vi "Arm Control Loop.vi"(8 "error in (no error)":errorcluster) -> ()   [LabVIEW 2011]
uses:
  Apendage State.ctl
  <vilib>/Rock Robotics/WPI/Solenoid/WPI_SolenoidValue.ctl
  Robot Global Data.vi
  <vilib>/Rock Robotics/WPI/Solenoid/WPI_SolenoidSetEnum.vi
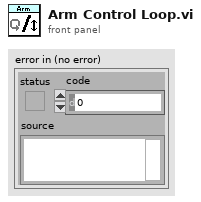
[diagram p1: front panel]
types:
  T1 = typedef "WPI_SolenoidValue.ctl" = enum16{"Off", "On", "Forward", "Reverse"}
  T2 = typedef "Apendage State.ctl" = enum16{"Unknown", "Down", "Up"}
  T3 = typedef "WPI_SolenoidDevRef.ctl" = cluster{"DevStatus":errorcluster, "Solenoid Module":T4, "Forward Solenoid Channel":T5, "Reverse Solenoid Channel":T5}
  T4 = typedef "FPGA_TypedefSolenoidModule.ctl" = enum16{"Solenoid Module 1", "Solenoid Module 2"}
  T5 = typedef "WPI_SolenoidChannel.ctl" = enum8{"Solenoid 1", "Solenoid 2", "Solenoid 3", "Solenoid 4", "Solenoid 5", "Solenoid 6", "Solenoid 7", "Solenoid 8", "Invalid"}
  T6 = typedef "WPI_RelayDevRef.ctl" = cluster{"DevStatus":errorcluster, "Relay Channel":T7, "Digital Module":T8, "Relay Direction":T9}
  T7 = typedef "FPGA_DIORelayChannel.ctl" = enum8{"Relay 1", "Relay 2", "Relay 3", "Relay 4", "Relay 5", "Relay 6", "Relay 7", "Relay 8", "Invalid"}
  T8 = typedef "FPGA_TypedefDigitalModule.ctl" = enum16{"Digital Module 1", "Digital Module 2"}
  T9 = typedef "WPI_RelayDirection.ctl" = enum16{"Both directions", "Forward only", "Reverse only"}
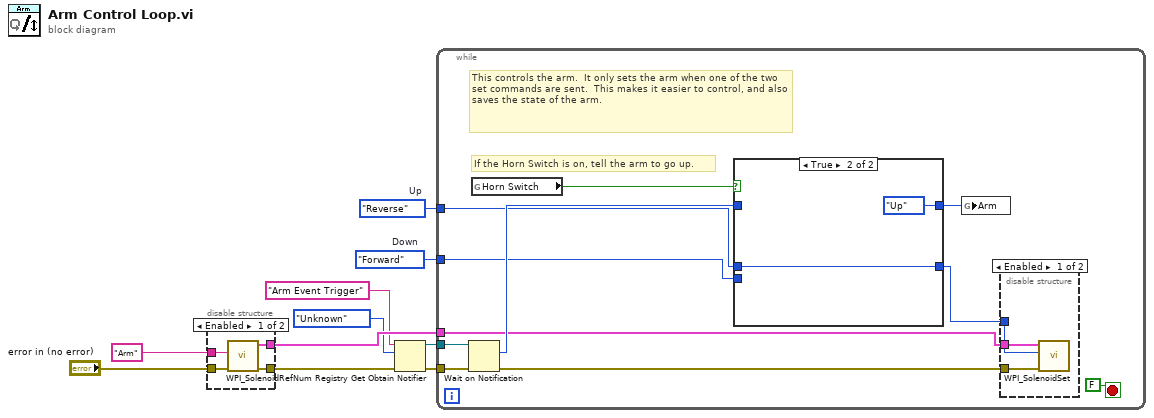
[diagram p0: block diagram]
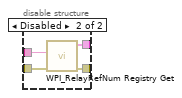
[diagram p2: hidden frame]
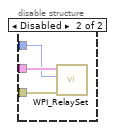
[diagram p3: hidden frame]
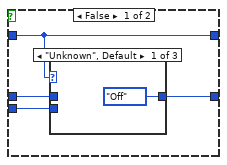
[diagram p4: hidden frame]
diagram:
  w1 = WPI_SolenoidValue."Forward"  # Down
  w2 = WPI_SolenoidValue."Reverse"  # Up
  n1 = disable-structure shown="Enabled" {
    disable-tunnel: [w14 w17] -> w8
    disable-tunnel: [w13 w18] -> w7
    disable-tunnel: "error in (no error)" -> [w12 w15]
    disable-tunnel: "Arm" ("refnum name") -> [w11 w16]
    frame Enabled {
      n2 = call <vilib>:"WPI_SolenoidRefNum Registry Get.vi"("error in (no error)"=w12, "refnum name"=w11) -> ("error out"=w13:errorcluster, "SolenoidDevRef"=w14:T3)  [unwired: 8 in]
    }
    frame Disabled {
      n3 = call <vilib>:"WPI_RelayRefNum Registry Get.vi"("error in (no error)"=w15, "refnum name"=w16) -> ("error out"=w18:errorcluster, "RelayDevRef"=w17:T6)  [unwired: 8 in]
    }
  }
  n4 = Obtain Notifier(name (unnamed)="Arm Event Trigger", notification data type=Apendage_State."Unknown", error in (no error)=w7) -> (notifier out=w10:refnum<notifier>, error out=w9:errorcluster)  [unwired: 1 in, 1 out]
  n5 = while {
    tunnel: w10 -> [w29]
    tunnel: w9 -> [w28]
    tunnel: w8 -> [w21]
    tunnel: w2 -> [w23]
    tunnel: w1 -> [w22]
    stop <- FALSE stop-if-true
    # "If the Horn Switch is on, tell the arm to go up."
    # "This controls the arm.  It only sets the arm when one of the two set commands are sent.  This makes it easier to control, and also saves the state of the arm."
    n6 = Wait on Notification(notifier=w29, error in (no error)=w28) -> (notification=w26:T2, error out=w19:errorcluster)  [unwired: 2 in, 2 out]
    n7 = global read "Robot Global Data.vi" "Horn Switch"() -> (w25:bool)
    n8 = case shown="True" w25 {
      tunnel: w26 -> [w39 _]
      tunnel: [w39 Apendage_State."Up"] -> w24
      tunnel: [w38 w43] -> w20
      tunnel: w23 -> [w37 w43]
      tunnel: w22 -> [w36 _]
      frame False {
        n9 = case shown="\"Unknown\", Default" w39 {
          tunnel: [WPI_SolenoidValue."Off" ("t") w41 w42] -> w38
          tunnel: w37 -> [_ _ w42]
          tunnel: w36 -> [_ w41 _]
          frame "Unknown", Default {
          }
          frame "Down" {
          }
          frame "Up" {
          }
        }
      }
      frame True {
      }
    }
    n10 = global write "Robot Global Data.vi" "Arm"(w24) -> ()
    n11 = disable-structure shown="Enabled" {
      disable-tunnel: w19 -> [w32 w34]
      disable-tunnel: w21 -> [w31 w35]
      disable-tunnel: w20 -> [w30 w33]
      frame Enabled {
        n12 = call-poly <vilib>:"WPI_SolenoidSet.vi"("error in (no error)"=w32, "Value"=w30, "SolenoidDevRef"=w31) -> ()  [unwired: 7 in, 2 out]
      }
      frame Disabled {
        n13 = call <vilib>:"WPI_RelaySet.vi"("error in (no error)"=w34, "RelayValue"=w33, "RelayDevRef"=w35) -> ()  [unwired: 7 in, 2 out]
      }
    }
  }
